vi "Unscale Booleans.vi"(8 "error in (no error)":errorcluster, 11 "Data Scaling in":refnum<class "Data Scaling.lvclass">) -> (0 "error out":errorcluster, 3 "Data Scaling out":refnum<class "Data Scaling.lvclass">)   [LabVIEW 2020, in "Unit Tests.lvlib" / "Data Scaling.lvclass"]
uses:
  Data Scaling.lvclass
  Frames & Messages/TypeDefs/Scaling Information.ctl
  <vilib>/addons/_JKI Toolkits/Caraya/classes/Test/Test.lvclass
  <vilib>/addons/_JKI Toolkits/Caraya/classes/Assert/Assert.lvclass
  BCI-1553 API.lvlib
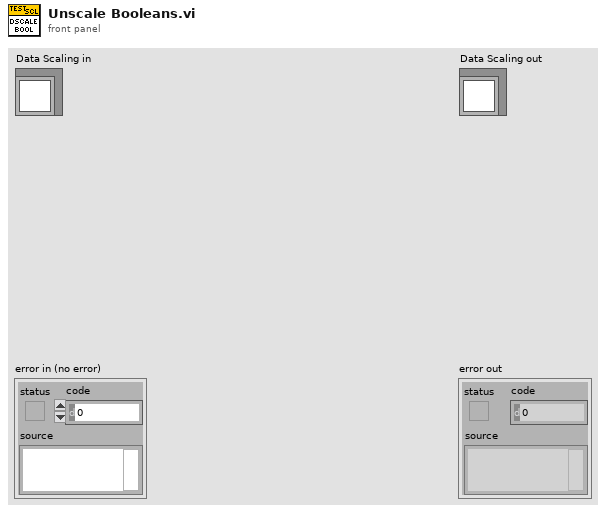
[diagram p1: front panel]
types:
  T1 = typedef "BCI-1553 API.lvlib/Scaling Information.ctl" = cluster{"Bit Offset":i32, "Bit Count":i32, "LSB Resolution":dbl, "2's Complement":bool, "Big Endian":bool, "Sign Bit":bool}
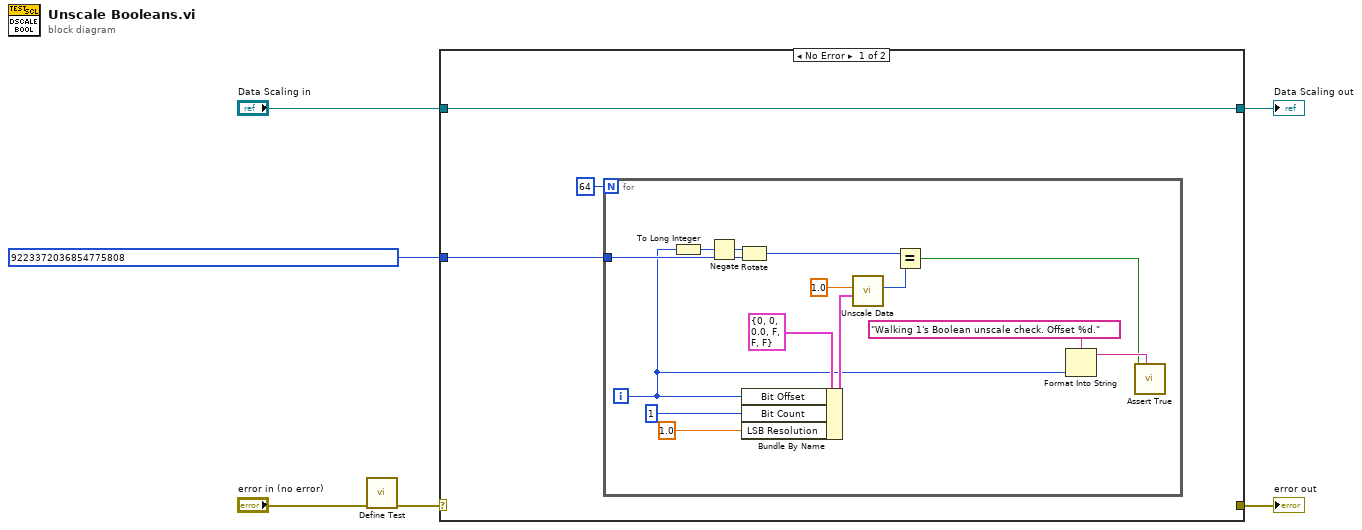
[diagram p0: block diagram]
diagram:
  n1 = call <vilib>:"Define Test.vi"("error in (no error)"="error in (no error)") -> ("error out"=w2:errorcluster)  [unwired: 9 in, 1 out]
  n2 = case shown="No Error" w2 {
    selector: w2 -> [_ w25]
    tunnel: [_ w25] -> w6
    tunnel: [w9 w24] -> w4
    tunnel: "Data Scaling in" -> [w9 w24]
    tunnel: u64 9223372036854775808 ("Raw Value") -> [w8 _]
    frame No Error {
      n3 = for {
        N: 64 -> [_]
        tunnel: w8 -> [w16]
        i -> [w11]
        n4 = To Long Integer(number=w11) -> (32bit integer=w17:i32)
        n5 = Negate(x=w17) -> (-x=w18:i32)
        n6 = Rotate(1:w16, 2:w18) -> (0:w15:u64)
        n7 = Bundle By Name(cluster=T1 {"Bit Offset"=0, "Bit Count"=0, "LSB Resolution"=0.0, "2's Complement"=FALSE, "Big Endian"=FALSE, "Sign Bit"=FALSE} ("Scaling Info"), "Bit Offset"=w11, "Bit Count"=1, "LSB Resolution"=1.0) -> (w20:T1)
        n8 = call "Unscale Data.vi"("Scaling Info"=w20, "Scaled Value"=1.0) -> ("Raw Value"=w14:u64)  [unwired: 8 in, 1 out]
        n9 = Equal?(x=w15, y=w14) -> (x = y?=w10:bool)
        n10 = Format Into String(format string="Walking 1's Boolean unscale check. Offset %d." ("Label"), w11) -> (resulting string=w12:string)  [unwired: 2 in, 1 out]
        n11 = call <vilib>:"Assert True.vi"("Label"=w12, "True?"=w10) -> ()  [unwired: 8 in, 2 out]
      }
    }
    frame Error {
    }
  }
  "error out" <- w6
  "Data Scaling out" <- w4
